vi "E441X_PM_Configure_Averaging.vi"(0 "VISA session":refnum<visa-resource-name>, 1 "Channel (0: A)":i32(ring) items=["A", "B"], 5 "State (T: On)":bool=TRUE, 7 "Filter Length (4)":i32=4, 11 "error in (no error)":errorcluster {"code" format="%.0x"}) -> (4 "dup VISA session":refnum<visa-resource-name>, 15 "error out":errorcluster {"code" format="%.0x"})   [LabVIEW 2015]
doc: "This VI configures the input averaging."
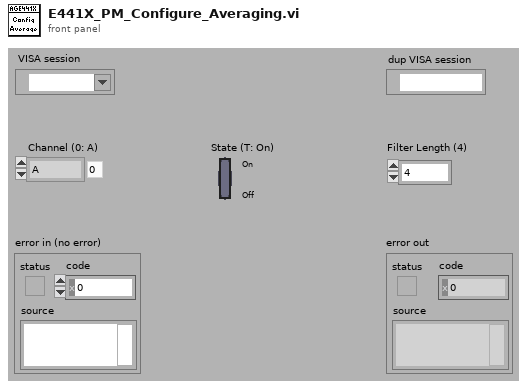
[diagram p1: front panel]
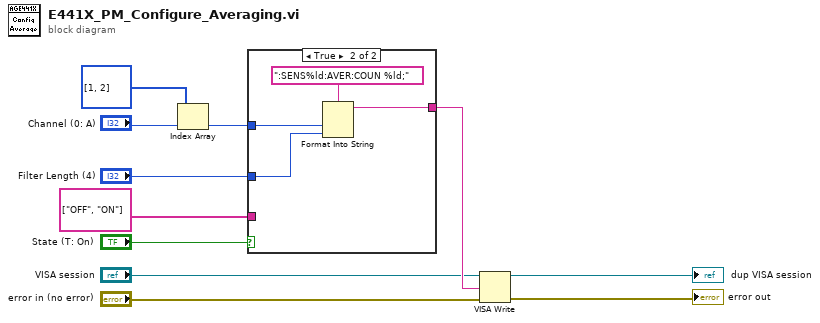
[diagram p0: block diagram]
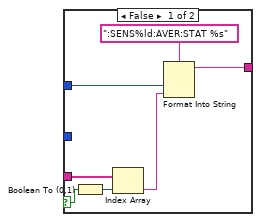
[diagram p2: hidden frame]
diagram:
  n1 = Index Array(array=i32[] [1, 2], index="Channel (0: A)") -> (element=w8:i32)
  n2 = case shown="True" "State (T: On)" {
    selector: "State (T: On)" -> [w16 _]
    tunnel: string[] ["OFF", "ON"] -> [w17 _]
    tunnel: w8 -> [w14 w21]
    tunnel: "Filter Length (4)" -> [_ w20]
    tunnel: [w12 w19] -> w5
    frame False {
      n3 = Boolean To (0,1)(Boolean=w16) -> (0, 1=w18:i16)
      n4 = Index Array(array=w17, index=w18) -> (element=w15:string)
      n5 = Format Into String(format string=":SENS%ld:AVER:STAT %s", w14, w15) -> (resulting string=w12:string)  [unwired: 2 in, 1 out]
    }
    frame True {
      n6 = Format Into String(format string=":SENS%ld:AVER:COUN %ld;", w21, w20) -> (resulting string=w19:string)  [unwired: 2 in, 1 out]
    }
  }
  n7 = VISA Write(VISA resource name="VISA session", write buffer=w5, error in (no error)="error in (no error)") -> (VISA resource name out=→"dup VISA session":refnum<visa-resource-name>, error out=→"error out":errorcluster)  [unwired: 1 out]
